vi "Read_raw_meas_setup.vi"(8 "Setup file string":string, 9 "Analysis Info cluster In":T1[](array[typedef]) {"Kurt_u" format="%_3g"; "u^4" format="%_3g"; "u^3" format="%_3g"; "Sd Error in Variance" format="%_3g"; "u^2" format="%_3g"; "Sd Error in Mean" format="%_3g"; "U" format="%_3g"; "Sync Delay Time (s)" format="%.4f"; "Total Meas Time (s)" format="%_5g"; "Skew_u" format="%_3g"; "% u'/U" format="%_3g"}) -> (0 "No of Blocks":i32=1, 1 "Time per Block (s)":dbl=100.0 format="%^_5g", 3 "Analysis Info clusterOut":T1[](array[typedef])=[{"Colour"=0, "Inst type"=enum."Pitot-static tube", "Inst name"="Manometer voltage", "Symbol"="U", "Code name"="", "Extra Info"="U", "Inst Array"=enum."PWA", "U"=0.0, "u^2"=0.0, "u^3"=0.0, "u^4"=0.0, "Skew_u"=0.0, "Kurt_u"=0.0, "Sd Error in Mean"=0.0, "% u'/U"=0.0, "X"=0.0, "Y"=0.0, "Z"=0.0, "Timescale integral Estimate"=0.0, "Sd Error in Variance"=0.0, "Calib File"=path "", "Calib Constants"=[], "Output Position"=FALSE, "Stats"=enum."None", "Av Sampling Rate"=0.0, "Av No of Samples"=0.0, "Total Meas Time (s)"=0.0, "OrigChName"="", "Max value"=0.0, "Min value"=0.0, "Req Sample Rate Hz"=0.0, "Sync Delay Time (s)"=0.0, "Ch No"=0, "Device"="", "Use Latest Calib"=FALSE, "Port"="", "Metadata Ch Names"=[], "Metadata Ch Values"=[], "Label"="", "chState"=enum."Solo", "Point Drift"=0.0, "inputConfig"=""}, {"Colour"=0, "Inst type"=enum."Pitot-static tube", "Inst name"="Manometer voltage", "Symbol"="U", "Code name"="", "Extra Info"="U", "Inst Array"=enum."PWA", "U"=0.0, "u^2"=0.0, "u^3"=0.0, "u^4"=0.0, "Skew_u"=0.0, "Kurt_u"=0.0, "Sd Error in Mean"=0.0, "% u'/U"=0.0, "X"=0.0, "Y"=0.0, "Z"=0.0, "Timescale integral Estimate"=0.0, "Sd Error in Variance"=0.0, "Calib File"=path "", "Calib Constants"=[], "Output Position"=FALSE, "Stats"=enum."None", "Av Sampling Rate"=0.0, "Av No of Samples"=0.0, "Total Meas Time (s)"=0.0, "OrigChName"="", "Max value"=0.0, "Min value"=0.0, "Req Sample Rate Hz"=0.0, "Sync Delay Time (s)"=0.0, "Ch No"=0, "Device"="", "Use Latest Calib"=FALSE, "Port"="", "Metadata Ch Names"=[], "Metadata Ch Values"=[], "Label"="", "chState"=enum."Solo", "Point Drift"=0.0, "inputConfig"=""}, {"Colour"=0, "Inst type"=enum."Pitot-static tube", "Inst name"="Manometer voltage", "Symbol"="U", "Code name"="", "Extra Info"="U", "Inst Array"=enum."PWA", "U"=0.0, "u^2"=0.0, "u^3"=0.0, "u^4"=0.0, "Skew_u"=0.0, "Kurt_u"=0.0, "Sd Error in Mean"=0.0, "% u'/U"=0.0, "X"=0.0, "Y"=0.0, "Z"=0.0, "Timescale integral Estimate"=0.0, "Sd Error in Variance"=0.0, "Calib File"=path "", "Calib Constants"=[], "Output Position"=FALSE, "Stats"=enum."None", "Av Sampling Rate"=0.0, "Av No of Samples"=0.0, "Total Meas Time (s)"=0.0, "OrigChName"="", "Max value"=0.0, "Min value"=0.0, "Req Sample Rate Hz"=0.0, "Sync Delay Time (s)"=0.0, "Ch No"=0, "Device"="", "Use Latest Calib"=FALSE, "Port"="", "Metadata Ch Names"=[], "Metadata Ch Values"=[], "Label"="", "chState"=enum."Solo", "Point Drift"=0.0, "inputConfig"=""}, {"Colour"=0, "Inst type"=enum."Pitot-static tube", "Inst name"="Manometer voltage", "Symbol"="U", "Code name"="", "Extra Info"="U", "Inst Array"=enum."PWA", "U"=0.0, "u^2"=0.0, "u^3"=0.0, "u^4"=0.0, "Skew_u"=0.0, "Kurt_u"=0.0, "Sd Error in Mean"=0.0, "% u'/U"=0.0, "X"=0.0, "Y"=0.0, "Z"=0.0, "Timescale integral Estimate"=0.0, "Sd Error in Variance"=0.0, "Calib File"=path "", "Calib Constants"=[], "Output Position"=FALSE, "Stats"=enum."None", "Av Sampling Rate"=0.0, "Av No of Samples"=0.0, "Total Meas Time (s)"=0.0, "OrigChName"="", "Max value"=0.0, "Min value"=0.0, "Req Sample Rate Hz"=0.0, "Sync Delay Time (s)"=0.0, "Ch No"=0, "Device"="", "Use Latest Calib"=FALSE, "Port"="", "Metadata Ch Names"=[], "Metadata Ch Values"=[], "Label"="", "chState"=enum."Solo", "Point Drift"=0.0, "inputConfig"=""}] {"Kurt_u" format="%_3g"; "u^4" format="%_3g"; "u^3" format="%_3g"; "Sd Error in Variance" format="%_3g"; "u^2" format="%_3g"; "Sd Error in Mean" format="%_3g"; "U" format="%_3g"; "Sync Delay Time (s)" format="%.4f"; "Total Meas Time (s)" format="%_5g"; "Skew_u" format="%_3g"; "% u'/U" format="%_3g"})   [LabVIEW 2022 SP3]
uses:
  Globals/Meas_global.vi
  Globals/Trav_pos_global.vi
  Globals/LDA_global.vi
  Controls/Inst_type.ctl
  Controls/Instrument_Array.ctl
  Controls/Analysis_info_cluster.ctl
  Controls/channelState.ctl
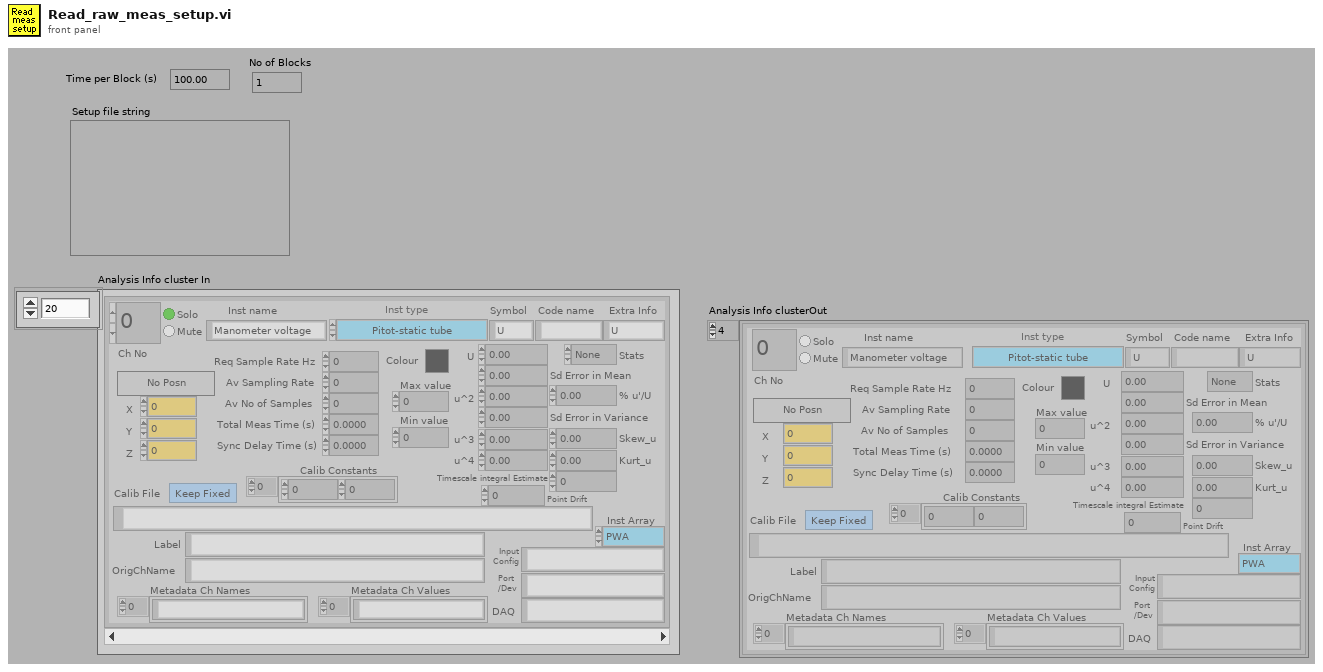
[diagram p1: front panel]
types:
  T1 = typedef "Analysis_info_cluster.ctl" = cluster{"Colour":u32, "Inst type":T2, "Inst name":string, "Symbol":string, "Code name":string, "Extra Info":string, "Inst Array":T3, "U":dbl, "u^2":dbl, "u^3":dbl, "u^4":dbl, "Skew_u":dbl, "Kurt_u":dbl, "Sd Error in Mean":dbl, "% u'/U":dbl, "X":dbl, "Y":dbl, "Z":dbl, "Timescale integral Estimate":dbl, "Sd Error in Variance":dbl, "Calib File":path, "Calib Constants":dbl[], "Output Position":bool, "Stats":enum16{"None", "Basic", "Full"}, "Av Sampling Rate":dbl, "Av No of Samples":dbl, "Total Meas Time (s)":dbl, "OrigChName":string, "Max value":dbl, "Min value":dbl, "Req Sample Rate Hz":dbl, "Sync Delay Time (s)":dbl, "Ch No":i16, "Device":string, "Use Latest Calib":bool, "Port":string, "Metadata Ch Names":string[], "Metadata Ch Values":string[], "Label":string, "chState":T4, "Point Drift":dbl, "inputConfig":string}
  T2 = typedef "Inst_type.ctl" = enum16{"Raw voltage", "Raw with zero offsetting", "Propeller anemometer", "Pressure Transducer", "Pitot-static tube", "Hot wire", "Cross wire 1", "Cross wire 2", "Generic Linear", "Generic Polynomial", "Generic BackPoly", "Fast FID", "Thermocouple", "Cold wire", "Pulsed Wire", "LDA Vel", "LDA Tran time", "LDA Arr time", "Microphone"}
  T3 = typedef "Instrument_Array.ctl" = enum16{"PWA", "LDA", "Analogue"}
  T4 = typedef "channelState.ctl" = enum32{"No Selection", "Solo", "Mute"}
  T5 = typedef "Post_Process.ctl" = enum16{"Take New Data", "Post Process Raw Data File"}
  T6 = enum16{"From String to Cluster", "From Cluster to String"}
  T7 = typedef "Graph_Type.ctl" = enum16{"Show no graph", "Voltage trace", "Velocity trace", "Vel histogram", "Spectrum", "f.E(f) v Log f", "Auto-Corr"}
  T8 = cluster{"Plot 1":u16, "Plot 2":u16, "Save graph":u16, "Plot Type":T7}
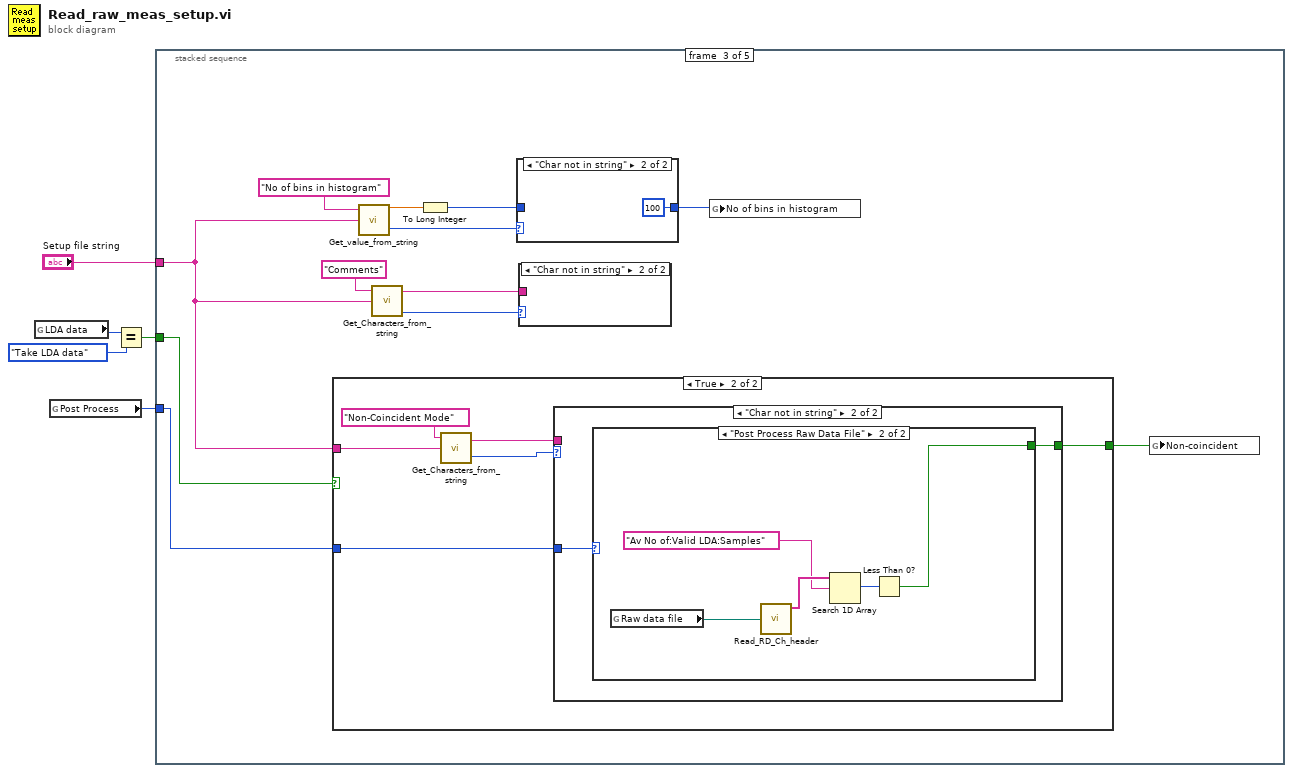
[diagram p0: block diagram]
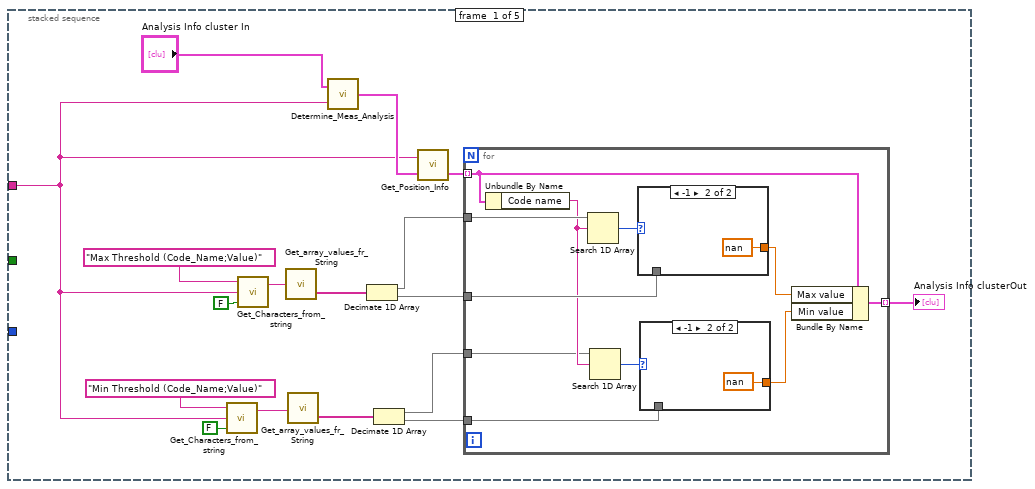
[diagram p2: hidden frame]
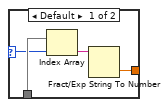
[diagram p3: hidden frame]
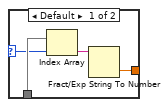
[diagram p4: hidden frame]
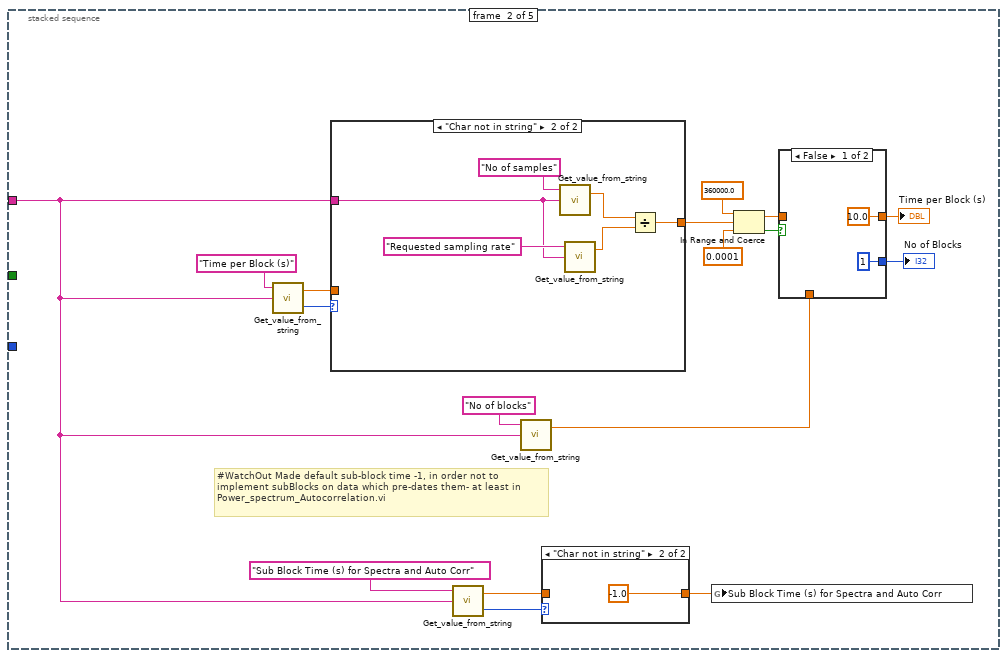
[diagram p5: hidden frame]
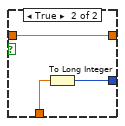
[diagram p6: hidden frame]
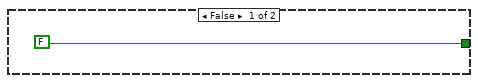
[diagram p9: hidden frame]
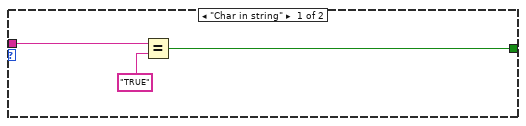
[diagram p10: hidden frame]
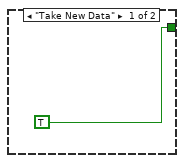
[diagram p11: hidden frame]
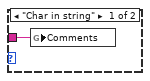
[diagram p12: hidden frame]
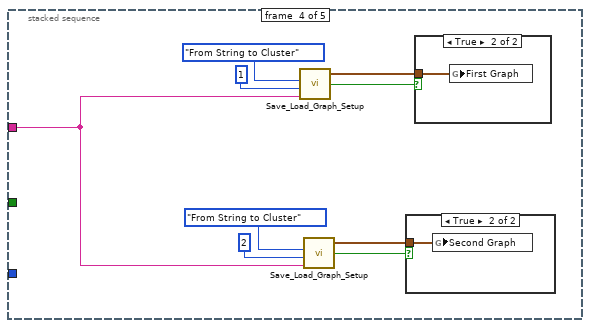
[diagram p14: hidden frame]
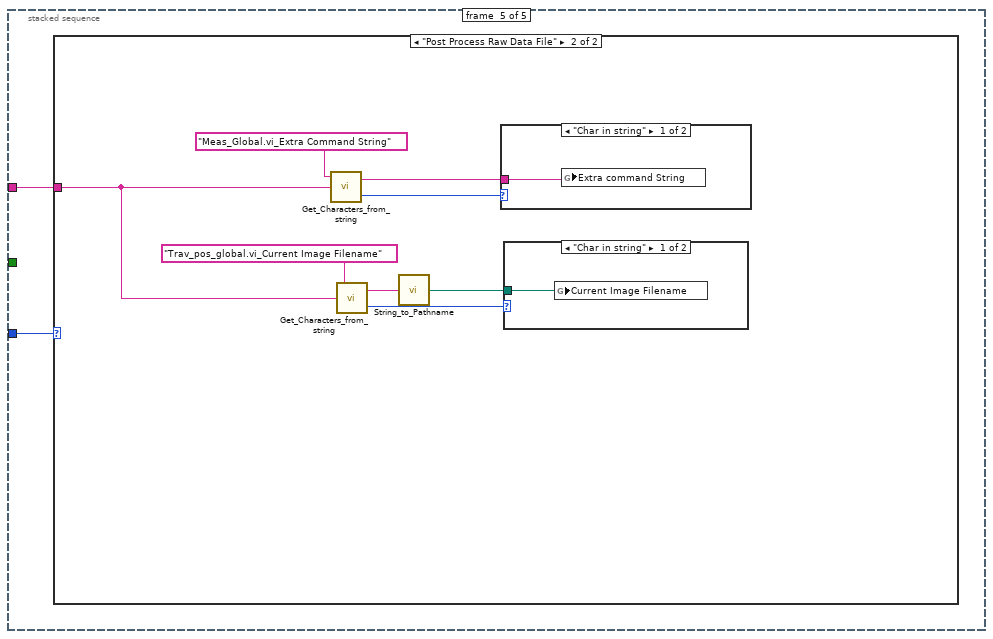
[diagram p17: hidden frame]
diagram:
  n1 = global read "Meas_global.vi" "LDA data"() -> (w3:enum16{"No LDA data", "Take LDA data"})
  n2 = global read "Meas_global.vi" "Post Process"() -> (w5:T5)
  n3 = Equal?(x=w3, y=enum16{"No LDA data", "Take LDA data"}."Take LDA data" ("LDA data")) -> (x = y?=w2:bool)
  n4 = stacked-sequence {
    tunnel: w5 -> [_ _ w75 _ w120]
    tunnel: w2 -> [_ _ w77 _ _]
    tunnel: "Setup file string" -> [w7 w55 w78 w108 w119]
    frame #0 {
      n5 = call "Get_Characters_from_string.vi"("Show Dialog?"=FALSE, "Input string"=w7, "Variable name"="Min Threshold (Code_Name;Value)") -> ("Value"=w14:string)  [unwired: 1 out]
      n6 = call "Get_Characters_from_string.vi"("Show Dialog?"=FALSE, "Input string"=w7, "Variable name"="Max Threshold (Code_Name;Value)") -> ("Value"=w16:string)  [unwired: 1 out]
      n7 = call "Get_array_values_fr_String.vi"("String Value"=w16) -> ("String array"=w13:string[])  [unwired: 1 out]
      n8 = call "Get_array_values_fr_String.vi"("String Value"=w14) -> ("String array"=w10:string[])  [unwired: 1 out]
      n9 = call "Determine_Meas_Analysis.vi"("Pre Setup String"=w7, "Analysis info Cluster In"="Analysis Info cluster In") -> ("Analysis info Cluster Out"=w22:T1[])
      n10 = Decimate 1D Array(w13) -> (w12:string[], w11:string[])
      n11 = Decimate 1D Array(w10) -> (w9:string[], w8:string[])
      n12 = call "Get_Position_Info.vi"("Analysis Info cluster"=w22, "Setup file string"=w7) -> ("Analysis Info cluster 2"=w17:T1[])  [unwired: 1 in]
      n13 = for {
        tunnel: w17 -> [w32] mode=indexing
        tunnel: w12 -> [w33]
        tunnel: [w31] -> w15 mode=indexing
        tunnel: w11 -> [w28]
        tunnel: w9 -> [w25]
        tunnel: w8 -> [w24]
        n14 = Unbundle By Name(w32) -> ("Code name"=w26:string)
        n15 = Search 1D Array(1D array=w33, element=w26) -> (index of element=w29:i32)  [unwired: 1 in]
        n16 = Search 1D Array(1D array=w25, element=w26) -> (index of element=w27:i32)  [unwired: 1 in]
        n17 = case shown="-1" w29 {
          selector: w29 -> [w39 _]
          tunnel: [w41 nan ("Max value")] -> w30
          tunnel: w28 -> [w40 _]
          frame Default {
            n18 = Index Array(array=w40, index=w39) -> (element=w42:string)
            n19 = Fract/Exp String To Number(string=w42) -> (number=w41:dbl)  [unwired: 3 in, 1 out]
          }
          frame -1 {
          }
        }
        n20 = case shown="-1" w27 {
          selector: w27 -> [w34 _]
          tunnel: [w36 nan ("Max value")] -> w23
          tunnel: w24 -> [w35 _]
          frame Default {
            n21 = Index Array(array=w35, index=w34) -> (element=w37:string)
            n22 = Fract/Exp String To Number(string=w37) -> (number=w36:dbl)  [unwired: 3 in, 1 out]
          }
          frame -1 {
          }
        }
        n23 = Bundle By Name(cluster=w32, "Max value"=w30, "Min value"=w23) -> (w31:T1)
      }
      "Analysis Info clusterOut" <- w15
    }
    frame #1 {
      # "#WatchOut Made default sub-block time -1, in order not to implement subBlocks on data which pre-dates them- at least in Power_spectrum_Autocorrelation.vi"
      n24 = call "Get_value_from_string.vi"("Input string"=w55, "Variable name"="Time per Block (s)") -> ("Status"=w58:enum16{"Char in string", "Char not in string"}, "Value"=w57:dbl)  [unwired: 1 in]
      n25 = case shown="\"Char not in string\"" w58 {
        tunnel: [w68 w69] -> w51
        tunnel: w57 -> [w68 _]
        tunnel: w55 -> [_ w72]
        frame "Char in string" {
        }
        frame "Char not in string" {
          n26 = call "Get_value_from_string.vi"("Input string"=w72, "Variable name"="No of samples") -> ("Value"=w71:dbl)  [unwired: 1 in, 1 out]
          n27 = call "Get_value_from_string.vi"("Input string"=w72, "Variable name"="Requested sampling rate") -> ("Value"=w70:dbl)  [unwired: 1 in, 1 out]
          n28 = Divide(x=w71, y=w70) -> (x/y=w69:dbl)
        }
      }
      n29 = call "Get_value_from_string.vi"("Input string"=w55, "Variable name"="Sub Block Time (s) for Spectra and Auto Corr") -> ("Status"=w53:enum16{"Char in string", "Char not in string"}, "Value"=w54:dbl)  [unwired: 1 in]
      n30 = call "Get_value_from_string.vi"("Input string"=w55, "Variable name"="No of blocks") -> ("Value"=w44:dbl)  [unwired: 1 in, 1 out]
      n31 = case shown="\"Char not in string\"" w53 {
        tunnel: w54 -> [w66 _]
        tunnel: [w66 -1.0 ("No of Sub Blocks for Spectra and Auto correlation")] -> w52
        frame "Char in string" {
        }
        frame "Char not in string" {
        }
      }
      n32 = global write "Meas_global.vi" "Sub Block Time (s) for Spectra and Auto Corr"(w52) -> ()
      n33 = In Range and Coerce(upper limit=360000.0, x=w51, lower limit=0.0001) -> (coerced(x)=w46:dbl, In Range?=w48:bool)
      n34 = case shown="False" w48 {
        tunnel: [10.0 ("upper limit") w65] -> w47
        tunnel: w46 -> [_ w65]
        tunnel: [1 w63] -> w45
        tunnel: w44 -> [_ w64]
        frame False {
        }
        frame True {
          n35 = To Long Integer(number=w64) -> (32bit integer=w63:i32)
        }
      }
      "No of Blocks" <- w45
      "Time per Block (s)" <- w47
    }
    frame #2 {
      n36 = case shown="True" w77 {
        tunnel: [FALSE w89] -> w76
        tunnel: w78 -> [_ w91]
        tunnel: w75 -> [_ w88]
        frame False {
        }
        frame True {
          n37 = call "Get_Characters_from_string.vi"("Input string"=w91, "Variable name"="Non-Coincident Mode" ("Pre Setup String")) -> ("Status"=w90:enum16{"Char in string", "Char not in string"}, "Value"=w92:string)  [unwired: 1 in]
          n38 = case shown="\"Char not in string\"" w90 {
            tunnel: w92 -> [w96 _]
            tunnel: [w94 w98] -> w89
            tunnel: w88 -> [_ w97]
            frame "Char in string" {
              n39 = Equal?(x=w96, y="TRUE") -> (x = y?=w94:bool)
            }
            frame "Char not in string" {
              n40 = case shown="\"Post Process Raw Data File\"" w97 {
                tunnel: [TRUE w100] -> w98
                frame "Take New Data" {
                }
                frame "Post Process Raw Data File" {
                  n41 = global read "Meas_global.vi" "Raw data file"() -> (w104:path)
                  n42 = call "Read_RD_Ch_header.vi"("Raw data file"=w104) -> ("Ch Name Out"=w103:string[])  [unwired: 3 out]
                  n43 = Search 1D Array(1D array=w103, element="Av No of:Valid LDA:Samples") -> (index of element=w101:i32)  [unwired: 1 in]
                  n44 = Less Than 0?(x=w101) -> (x < 0?=w100:bool)
                }
              }
            }
          }
        }
      }
      n45 = call "Get_value_from_string.vi"("Input string"=w78, "Variable name"="No of bins in histogram") -> ("Status"=w85:enum16{"Char in string", "Char not in string"}, "Value"=w84:dbl)  [unwired: 1 in]
      n46 = call "Get_Characters_from_string.vi"("Input string"=w78, "Variable name"="Comments") -> ("Status"=w82:enum16{"Char in string", "Char not in string"}, "Value"=w81:string)  [unwired: 1 in]
      n47 = To Long Integer(number=w84) -> (32bit integer=w83:i32)
      n48 = case shown="\"Char not in string\"" w85 {
        tunnel: w83 -> [w106 _]
        tunnel: [w106 100] -> w79
        frame "Char in string" {
        }
        frame "Char not in string" {
        }
      }
      n49 = case shown="\"Char not in string\"" w82 {
        tunnel: w81 -> [w105 _]
        frame "Char in string" {
          n50 = global write "Meas_global.vi" "Comments"(w105) -> ()
        }
        frame "Char not in string" {
        }
      }
      n51 = global write "Meas_global.vi" "No of bins in histogram"(w79) -> ()
      n52 = global write "LDA_global.vi" "Non-coincident"(w76) -> ()
    }
    frame #3 {
      n53 = call "Save_Load_Graph_Setup.vi"("Setup String in"=w108, "Graph Number"=1, "Mode"=T6."From String to Cluster") -> ("Variables found?"=w114:bool, "Graph Out"=w113:T8)  [unwired: 1 in, 1 out]
      n54 = call "Save_Load_Graph_Setup.vi"("Setup String in"=w108, "Graph Number"=2, "Mode"=T6."From String to Cluster") -> ("Variables found?"=w110:bool, "Graph Out"=w109:T8)  [unwired: 1 in, 1 out]
      n55 = case shown="True" w110 {
        tunnel: w109 -> [_ w117]
        frame False {
        }
        frame True {
          n56 = global write "Meas_global.vi" "Second Graph"(w117) -> ()
        }
      }
      n57 = case shown="True" w114 {
        tunnel: w113 -> [_ w118]
        frame False {
        }
        frame True {
          n58 = global write "Meas_global.vi" "First Graph"(w118) -> ()
        }
      }
    }
    frame #4 {
      n59 = case shown="\"Post Process Raw Data File\"" w120 {
        tunnel: w119 -> [_ w126]
        frame "Take New Data" {
        }
        frame "Post Process Raw Data File" {
          n60 = call "Get_Characters_from_string.vi"("Input string"=w126, "Variable name"="Meas_Global.vi_Extra Command String" ("Label for characters")) -> ("Status"=w121:enum16{"Char in string", "Char not in string"}, "Value"=w122:string)  [unwired: 1 in]
          n61 = call "Get_Characters_from_string.vi"("Input string"=w126, "Variable name"="Trav_pos_global.vi_Current Image Filename" ("Label for characters")) -> ("Status"=w123:enum16{"Char in string", "Char not in string"}, "Value"=w125:string)  [unwired: 1 in]
          n62 = call "String_to_Pathname.vi"("Input String"=w125) -> ("path"=w124:path)
          n63 = case shown="\"Char in string\"" w121 {
            tunnel: w122 -> [w129 _]
            frame "Char in string" {
              n64 = global write "Meas_global.vi" "Extra command String"(w129) -> ()
            }
            frame "Char not in string" {
            }
          }
          n65 = case shown="\"Char in string\"" w123 {
            tunnel: w124 -> [w130 _]
            frame "Char in string" {
              n66 = global write "Trav_pos_global.vi" "Current Image Filename"(w130) -> ()
            }
            frame "Char not in string" {
            }
          }
        }
      }
    }
  }
